vi "Change_Client.vi"(8 "错误输入（无错误）":errorcluster, 11 "设备信息":T1) -> (0 "错误输出":errorcluster)   [LabVIEW 2020]
panel:
  # "嗯嗯"
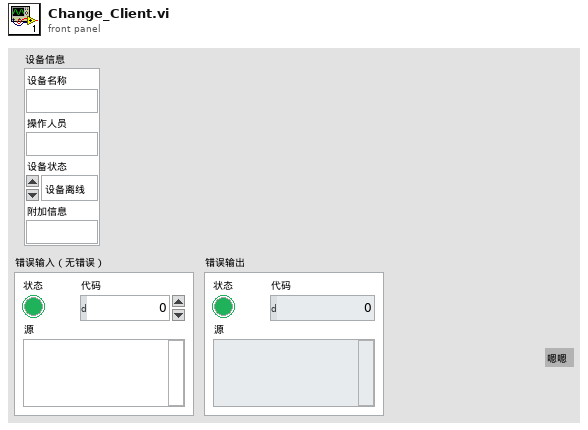
[diagram p1: front panel]
types:
  T1 = cluster{"设备名称":string, "操作人员":string, "设备状态":enum16{"设备离线", "设备正常", "设备缺料", "设备故障", "质量报警"}, "附加信息":string}
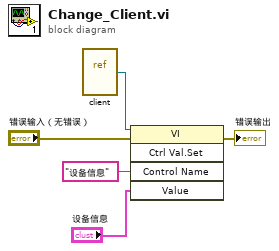
[diagram p0: block diagram]
diagram:
  n1 = vi-ref "client.vi"() -> (w5:refnum<vi>)
  n2 = invoke class="VI" method="Ctrl Val.Set"(reference=w5, error in="错误输入（无错误）", "Control Name"="设备信息" ("控件名"), "Value"="设备信息") -> (error out=→"错误输出":errorcluster)  [unwired: 1 in, 4 out]
